vi "Get External Channel Refs.vi"(8 "error in (no error)":errorcluster, 9 "Triggers":T1[](array[typedef]), 10 "Internal Triggers":cluster{"Chan Refs":T2[], "Prev. Values":dbl[]} {"Chan Refs" format="%.0x"}, 11 "Device Ref in":T4 format="%.0x") -> (0 "error out":errorcluster, 2 "Refs":T3 {"Channels" format="%.0x"; "Triggers" format="%.0x"}, 3 "Item Ref out":T4 format="%.0x")   [LabVIEW 2013, in "Instrument Addon System Explorer.lvlib"]
uses:
  Instrument Addon System Explorer.lvlib
  <vilib>/NI Veristand/Custom Device API/Custom Device Item Ref.ctl
  Shared/Types/External Trigger Refs.ctl
  <vilib>/NI Veristand/Custom Device API/Data Reference.ctl
  Shared/Types/Trigger Parameters.ctl
  <vilib>/NI Veristand/Custom Device API/Data Access Type.ctl
  <vilib>/NI Veristand/Custom Device API/Custom Device API.lvlib
  <vilib>/NI Veristand/Custom Device Tools/Custom Device Utility Library/Custom Device Utility Library.lvlib
  Shared/Instrument Addon Shared.lvlib
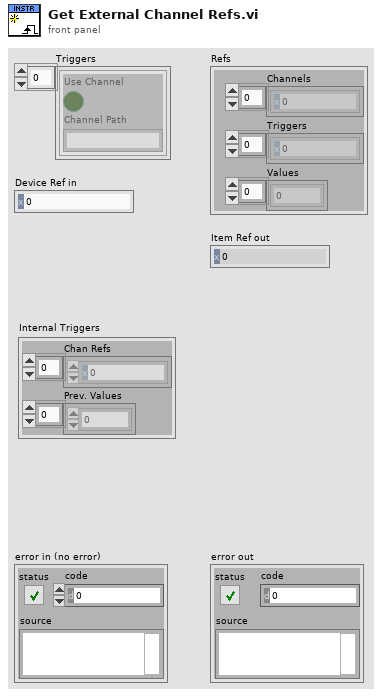
[diagram p1: front panel]
types:
  T1 = typedef "Instrument Addon Shared.lvlib/Trigger Parameters.ctl" = cluster{"Use Channel":bool, "Channel Path":string}
  T2 = typedef "Custom Device API.lvlib/Data Reference.ctl" = i32
  T3 = typedef "Instrument Addon Shared.lvlib/External Trigger Refs.ctl" = cluster{"Channels":T2[], "Triggers":T2[], "Values":dbl[]}
  T4 = typedef "Custom Device API.lvlib/Custom Device Item Ref.ctl" = u64
  T5 = typedef "Custom Device API.lvlib/Data Access Type.ctl" = enum16{"Read", "Write"}
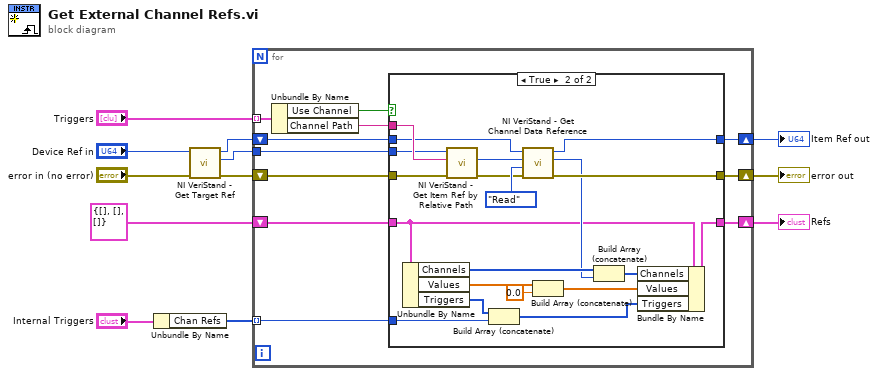
[diagram p0: block diagram]
diagram:
  n1 = Unbundle By Name("Internal Triggers") -> ("Chan Refs"=w3:T2[])
  n2 = call <vilib>:"NI VeriStand - Get Target Ref.vi"("error in"="error in (no error)", "Item Ref in"="Device Ref in") -> ("error out"=w5:errorcluster, "Target Ref"=w4:T4, "Item Ref out"=w6:T4)  [unwired: 6 in, 1 out]
  n3 = for {
    tunnel: "Triggers" -> [w23] mode=indexing
    tunnel: w3 -> [w22] mode=indexing
    tunnel: w4 -> [w21]
    shift-right: [w18] -> w10
    shift-left: w5 -> [w19]
    shift-right: [w16] -> w9
    shift-left: w6 -> [w17]
    shift-right: [w13] -> w7
    shift-left: T3 {"Channels"=[], "Triggers"=[], "Values"=[]} ("output cluster") -> [w14]
    n4 = Unbundle By Name(w23) -> ("Use Channel"=w15:bool, "Channel Path"=w20:string)
    n5 = case shown="True" w15 {
      tunnel: w22 -> [_ w35]
      tunnel: w21 -> [_ w45]
      tunnel: w20 -> [_ w46]
      tunnel: w19 -> [w26 w44]
      tunnel: [w26 w38] -> w18
      tunnel: w17 -> [w25 w42]
      tunnel: [w25 w41] -> w16
      tunnel: w14 -> [w24 w32]
      tunnel: [w24 w29] -> w13
      frame False {
      }
      frame True {
        n6 = Unbundle By Name(w32) -> ("Channels"=w37:T2[], "Values"=w34:dbl[], "Triggers"=w27:T2[])
        n7 = call <vilib>:"NI VeriStand - Get Item Ref by Relative Path.vi"("error in"=w44, "Relative Item Path"=w46, "Section Ref in"=w45) -> ("error out"=w39:errorcluster, "Item Ref"=w43:T4)  [unwired: 5 in, 2 out]
        n8 = Build Array (concatenate)(w27, w35) -> (w28:T2[])
        n9 = call <vilib>:"NI VeriStand - Get Channel Data Reference.vi"("error in (no error)"=w39, "Access"=Data_Access_Type."Read", "Channel Ref in"=w43, "Device Ref in"=w42) -> ("error out"=w38:errorcluster, "Channel Data Reference"=w36:T2, "Device Ref out"=w41:T4)  [unwired: 5 in]
        n10 = Build Array (concatenate)(w34, 0.0) -> (w30:dbl[])
        n11 = Build Array (concatenate)(w37, w36) -> (w31:T2[])
        n12 = Bundle By Name(cluster=w32, "Channels"=w31, "Values"=w30, "Triggers"=w28) -> (w29:T3)
      }
    }
  }
  "error out" <- w10
  "Item Ref out" <- w9
  "Refs" <- w7
